vi "FTW-SEQ-AddLast.vi"(1 "Add Last in Sequence":string, 3 "Sequencer":refnum<class "FTW-Sequencer.lvclass">) -> (0 "Sequencer out":refnum<class "FTW-Sequencer.lvclass">)   [LabVIEW 2013, in "FTW-Sequencer.lvclass"]
uses:
  FTW-Sequencer.lvclass
  FTW-Sequencer.lvclass/FTW-Sequencer.ctl
panel:
  # "Inputs"
  # "Outputs"
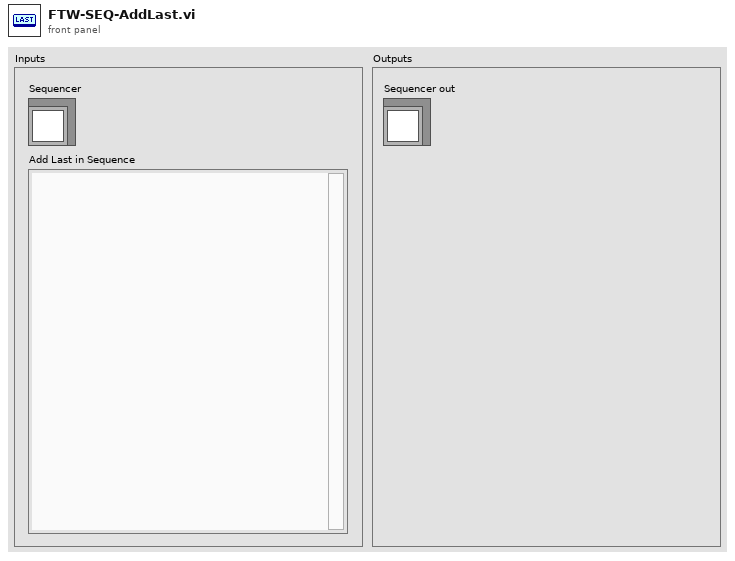
[diagram p1: front panel]
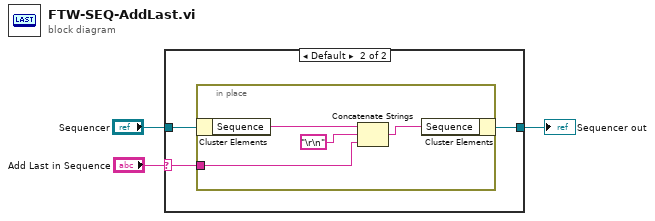
[diagram p0: block diagram]
diagram:
  n1 = case shown="Default" "Add Last in Sequence" {
    selector: "Add Last in Sequence" -> [_ w5]
    tunnel: "Sequencer" -> [w4 w7]
    tunnel: [w4 w6] -> w2
    frame "" {
    }
    frame Default {
      n2 = in-place {
        in-place-border: w5 -> [w8]
        n3 = in-place-cluster #1(w7) -> ("Sequence"=w9:string)
        n4 = Concatenate Strings(w9, "\r\n", w8) -> (w10:string)
        n5 = in-place-cluster #1("Sequence"=w10) -> (w6:refnum<class "FTW-Sequencer.lvclass">)
      }
    }
  }
  "Sequencer out" <- w2
